vi "Charger_Monitor.vi"(6 "Stop Refnum":refnum<vi>, 7 "Status Refnum":T1, 8 "error in":errorcluster, 10 "Index":i32) -> (0 "error out":errorcluster, 4 "done":bool)   [LabVIEW 2020]
uses:
  Charger_Status Refnum.ctl
  Drivers/Charger Test Set/Charger_Input Control.ctl
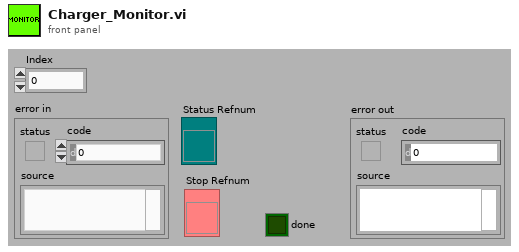
[diagram p1: front panel]
types:
  T1 = typedef "Charger_Status Refnum.ctl" = refnum<vi>
  T2 = typedef "Charger_Input Control.ctl" = cluster{"address":refnum<visa-resource-name>, "position":i32, "setpoint":dbl}
  T3 = typedef "MICS_Input Control.ctl" = cluster{"address":refnum<visa-resource-name>, "chan":u16, "ID":u32}
  T4 = typedef "Charger_States_Control.ctl" = enum16{"Enable", "Disable", "Adjust", "Pause", "na"}
  T5 = cluster{"MICS ID":u32, "VBAT":dbl, "ChargingState":string, "VBAT Slide":dbl, "Status":string, "TemperatureLevel":dbl, "IPG_ReceivedLevel":dbl, "VBAT Target":dbl, "Charger Setpoint":dbl, "Index":i32, "Ready":bool, "Charger Inputs":T2, "MICS Inputs":cluster{"address":refnum<visa-resource-name>, "chan":u16, "ID":u32}}
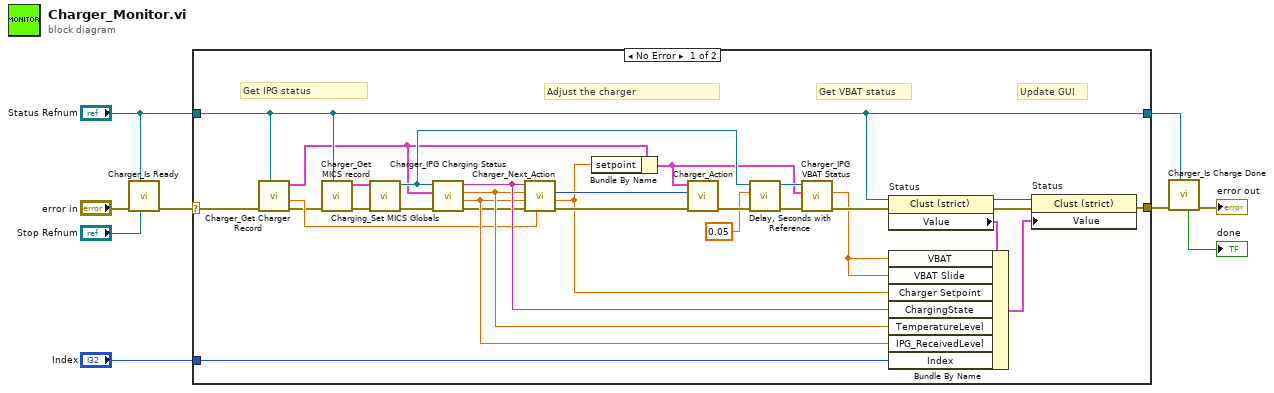
[diagram p0: block diagram]
diagram:
  n1 = call "Charger_Is Ready.vi"("Stop Refnum"="Stop Refnum", "Status Refnum"="Status Refnum", "error in"="error in") -> ("error out"=w7:errorcluster)  [unwired: 7 in, 1 out]
  n2 = case shown="No Error" w7 {
    selector: w7 -> [w25 w40]
    tunnel: [w31 w40] -> w3
    tunnel: "Status Refnum" -> [w12 w39]
    tunnel: "Index" -> [w30 _]
    tunnel: [w12 w39] -> w1
    frame No Error {
      # "Get VBAT status"
      # "Adjust the charger"
      # "Get IPG status"
      # "Update GUI"
      n3 = call "Charger_Get Charger Record.vi"("Status Refnum"=w12, "error in"=w25) -> ("error out"=w24:errorcluster, "Charger Setpoint"=w26:dbl, "Charger Inputs"=w11:T2)  [unwired: 3 in, 2 out]
      n4 = call "Charger_Get MICS record.vi"("Status Refnum"=w12, "error in"=w24) -> ("error out"=w27:errorcluster, "MICS Inputs"=w29:T3)  [unwired: 3 in, 3 out]
      n5 = call "Charging_Set MICS Globals.vi"("error in"=w27, "MICS inputs"=w29) -> ("error out"=w28:errorcluster, "address"=w15:refnum<visa-resource-name>)  [unwired: 4 in]
      n6 = call "Charger_IPG Charging Status.vi"("error in"=w28, "Charger Inputs"=w11, "MICS Dongle Address"=w15) -> ("error out"=w34:errorcluster, "IPG_ReceivedLevel"=w36:dbl, "TemperatureLevel"=w37:dbl, "ChargingState"=w38:string)  [unwired: 5 in]
      n7 = call "Charger_Next_Action.vi"("Setpoint"=w26, "error in"=w34, "ReceivedLevel"=w36, "Temperature"=w37, "ChargingState"=w38) -> ("error out"=w33:errorcluster, "Adjustment"=w19:dbl, "Charger"=w32:T4)  [unwired: 1 in, 1 out]
      n8 = Bundle By Name(cluster=w11, "setpoint"=w19) -> (w10:T2)
      n9 = call "Charger_Action.vi"("error in"=w33, "Operation"=w32, "Charger"=w10) -> ("error out"=w16:errorcluster)  [unwired: 6 in]
      n10 = call "Delay, Seconds with Reference.vi"("error in"=w16, "delay"=dbl[unit] 0.05, "VISA resource"=w15) -> ("error out"=w17:errorcluster, "VISA resource dup"=w14:refnum<visa-resource-name>)  [unwired: 3 in, 1 out]
      n11 = call "Charger_IPG VBAT Status.vi"("error in"=w17, "Charger Inputs"=w10, "MICS Dongle Address"=w14) -> ("error out"=w23:errorcluster, "VBAT"=w18:dbl)  [unwired: 6 in, 1 out]
      n12 = property on="Status" class="Clust (strict)"(reference=w12, error in=w23) -> (reference out=w20:T1, error out=w22:errorcluster, "Value"=w21:T5)
      n13 = Bundle By Name(cluster=w21, "VBAT"=w18, "VBAT Slide"=w18, "Charger Setpoint"=w19, "ChargingState"=w38, "TemperatureLevel"=w37, "IPG_ReceivedLevel"=w36, "Index"=w30) -> (w35:T5)
      n14 = property on="Status" class="Clust (strict)"(reference=w20, error in=w22, "Value"=w35) -> (error out=w31:errorcluster)  [unwired: 1 out]
    }
    frame Error {
    }
  }
  n15 = call "Charger_Is Charge Done.vi"("Status Refnum"=w1, "error in"=w3) -> ("error out"=→"error out":errorcluster, "done"=→"done":bool)  [unwired: 8 in]
